vi "dfd_SOS_Direct_IIR_I_C.vi"() -> ()   [LabVIEW 2017, in "NI_DigFilterTemp.lvlib"]
uses:
  <vilib>/addons/Digital Filter Design/NI_DigFilterTemp.lvlib
panel:
  in  "String":string="\n\n/* ---- Constants ----*/\n#define %CapName%_N_SECTIONS %kSection%\n#define %CapName%_N_XSTATES (2*%CapName%_N_SECTIONS)\n#define %CapName%_N_YSTATES (2*%CapName%_N_SECTIONS)\n#define %CapName%_N_STATES (%CapName%_N_XSTATES + %CapName%_N_YSTATES)\n#define %CapName%_N_COEFA (2*%CapName%_N_SECTIONS)\n#define %CapName%_N_COEFB (3*%CapName%_N_SECTIONS)\n\n/* ---- Global Variables Declaration ----*/\nstatic %CoefAType% %FilterBlkName%_CoefA[%CapName%_N_COEFA];\nstatic %CoefBType% %FilterBlkName%_CoefB[%CapName%_N_COEFB];\n%InternalFunctionsDeclaration%\n\n%ShiftDefine%\n\n%AssistantFunctions%\n\n/* ---- Implement the Fixed-Point Filter ---- */\n%OutType% %FilterBlkName%_Filtering (%InType% sampleIn, %FilterBlkName%_State state)\n{\n\tI32 accA, accB;\n\t%FilterBlkName%_State xstate = state;\n\t%FilterBlkName%_State ystate = state + %CapName%_N_XSTATES;\n\tint i;\n\tint iA, iB;\n\n\taccB = (%I32TypeCast%sampleIn << IN2SUM);\n\n\tiA = iB = 0;\n\tfor (i=0; i < %CapName%_N_SECTIONS; i++, iA+=2)\n\t{\n\t\t/* Filtering */\n\t\taccA = (%FilterBlkName%_%MultB%(%PreMultCast%(accB << SUM2MULT), %FilterBlkName%_CoefB[iB++]) << PROD2SUM);\n\t\taccA += (%FilterBlkName%_%MultB%(xstate[iA], %FilterBlkName%_CoefB[iB++]) << PROD2SUM);\n\t\taccA += (%FilterBlkName%_%MultB%(xstate[iA+1], %FilterBlkName%_CoefB[iB++]) << PROD2SUM);\n\t\taccA -= (%FilterBlkName%_%MultA%(ystate[iA], %FilterBlkName%_CoefA[iA]) << PROD2SUM);\n\t\taccA -= (%FilterBlkName%_%MultA%(ystate[iA+1], %FilterBlkName%_CoefA[iA+1]) << PROD2SUM);\n\n\t\t/* Update the internal states */\n\t\txstate[iA+1] = xstate[iA];\n\t\txstate[iA] = %PreMultCast%((accB << SUM2DELAY) << DELAY2MULT);\n\n\t\tystate[iA+1] = ystate[iA];\n\t\tystate[iA] = %PreMultCast%((accA << SUM2DELAY) << DELAY2MULT);\n\n\t\taccB = accA;\n\t}\n\n\t%ApplyGainAccA%\n\n\treturn (%OutType%)accA;\n}\n\n/* ---- Internal Functions ---- */\n%InternalFunctions%\n\n/* ---- Filter Coefficients ---- */\nstatic %CoefAType% %FilterBlkName%_CoefA [] = {\n%CoefficientsA%\n};\nstatic %CoefBType% %FilterBlkName%_CoefB [] = {\n%CoefficientsB%\n};\n"
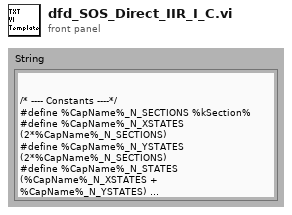
[diagram p1: front panel]
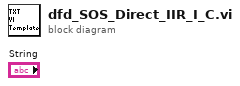
[diagram p0: block diagram]
diagram:
